vi "IMAQdx_AbsImage_Chameleon3_v5.vi"() -> ()   [LabVIEW 2015]
doc: "Take a single PixelFly exposure and display the result as an intensity graph.This VI illustrates the basics of taking an exposure with the PixelFly camera. Use Ctrl-H to get help on any of the controls\n\nCopyright 2001, The Cooke Corporation."
uses:
  Shared Libraries/Controls/FileName_Cluster.ctl
  <vilib>/userdefined/High Color/IMAQdx.ctl
  <vilib>/vision/driver/IMAQdx.llb/IMAQdx Acquisition Mode.ctl
  Shared Libraries/Controls/FileInfo_Global.vi
  <vilib>/vision/driver/NI_Vision_Acquisition_Software.lvlib
panel:
  out "DDE Done":bool=TRUE
  out "Waiting for PIXIS file":bool=TRUE
  in  "Flea Acquire":bool=TRUE
  in  "PIXIS Acquire":bool
  out "PIXIS Loop":i32
  out "CycleDone":bool
  out "PIXIS Frames":i64
  in  "Interrupt":bool
  out "Status":string="Running..."
  in  "stop":bool
  in  "Tab Control":enum32{"Setup", "Images", "Hardware status"}(tab)
  in  "PIXIS Data Series Name":string="PIXIS_Seq"
  in  "PointGrey File Parameters":T1={"Data Root"=path "D:/Data", "Index"=0, "Instrument"="Chameleon3"} {"Index" format="%04d"}
  in  "PIXIS Wave Name":string="Test_Img"
  out "PIXIS Image Note":string
  in  "Source of Control Data":refnum<k21>
  out "SPE delete path":path
  in  "PG Data Series Name":string="Chameleon3"
  in  "Camera Name":T2="Chameleon3"
  in  "Experiment":enum16{"Cs"}(ring)=4
  in  "Accept parameters from remote system":bool
  in  "PointGrey Magnification":dbl=1.0
  in  "Flea Image direction":enum16{"XY", "XZ"}(ring)=enum."XZ"
  in  "Flea Imaging technique":enum16{"Absorption", "Fluorescence", "RawImage"}(ring)
  in  "Send PG data to Igor?":bool
  out "Command to Igor":string
  out "Image note":string
  in  "PointGrey Wave Name":string="Chameleon3_Img"
  in  "Save files to archive?":bool
  out "Timeout":bool
  out "Trigger Overrun":bool
  in  "Source of File Data":refnum<k21>="\\\\Control\\VariableLibrary\\Instruction String"
  in  "Timeout (ms)":u32=20000
  in  "Gain":dbl
  in  "Shutter speed":dbl=100.0
  in  "PIXIS Magnification":dbl=1.0
  in  "PIXIS Image direction":enum16{"XY", "XZ"}(ring)
  in  "PIXIS Imaging technique":enum16{"Absorption", "Fluorescence", "RawImage"}(ring)
  in  "SPE File Path":path
  in  "Send PIXIS data to Igor?":bool
  in  "PIXIS File Parameters":T1={"Data Root"=path "I:/Data", "Index"=0, "Instrument"="PIXIS"} {"Index" format="%04d"}
  in  "Source of Wavemeter Data":refnum<k21>
  in  "Accept wavelength from remote system":bool
  in  "Flea Raw image to view":u16(ring)=1 items=["Clear", "Absorbtion", "Probe", "Background"]
  in  "Update Graphics":bool=TRUE
  out "Flea Raw Image":u16[][](graph)
  out "Flea Processed Image":sgl[][](graph)
  out "PIXIS Processed Image":sgl[][](graph)
  out "PIXIS Raw Image":u16[][](graph)
  in  "PIXIS Raw image to view":u16(ring)=1 items=["Clear", "Absorbtion", "Probe", "Background"]
  out "Camera Error":errorcluster
  out "DDE Error":errorcluster={"status"=FALSE, "code"=0, "source"="DDE Close: No Error"}
  out "Status Array":T3(array[cluster])
  in  "SPE Load Error In":errorcluster
  out "DataBlock Info":T4={"frame count"=4, "frame size"=524288, "frame stride"=524288, "N ROI"=1, "ROI widths"=[512], "ROI heights"=[512], "ROI sizes"=[524288], "ROI strides"=[524288]}
  out "DS Error":errorcluster
  out "XML Parse Errors":string
  out "Data Array Size":i32=1
  out "SPE Load Error Out":errorcluster
  out "Flea Path":path=path "D:/Data/Chameleon3temp.ibw"
  out "PIXIS Path":path=path "C:/Experiment/Data/PIXIStemp.ibw"
  out "PIXIS Images":u16[][][](array[numeric])
  out "Flea Images":u16[][][](array[numeric])
  out "Buffer Number":u32=1
  out "Flea Frames":i32
  out "Flea Loop":i32
  # "Image Acquisition v4.6 (FOR USB3 CAMERAS ONLY!!!)"
  # "Experimental Parameters"
  # "These are only get set on 1st run.\nUse a Gain of 0, Shutter Speed not used"
  # "In both techniques 3 images\nare aquired, but in Fluorescense\nthe 3rd is discarded"
  # "Obsolete: (now done with network variables)\nWhen paramaters are accepted from a remote system a DataSockets server\nmust be running on this machine (in start menu in National Instruments folder)"
  # "Camera configuration"
  # "File configuration"
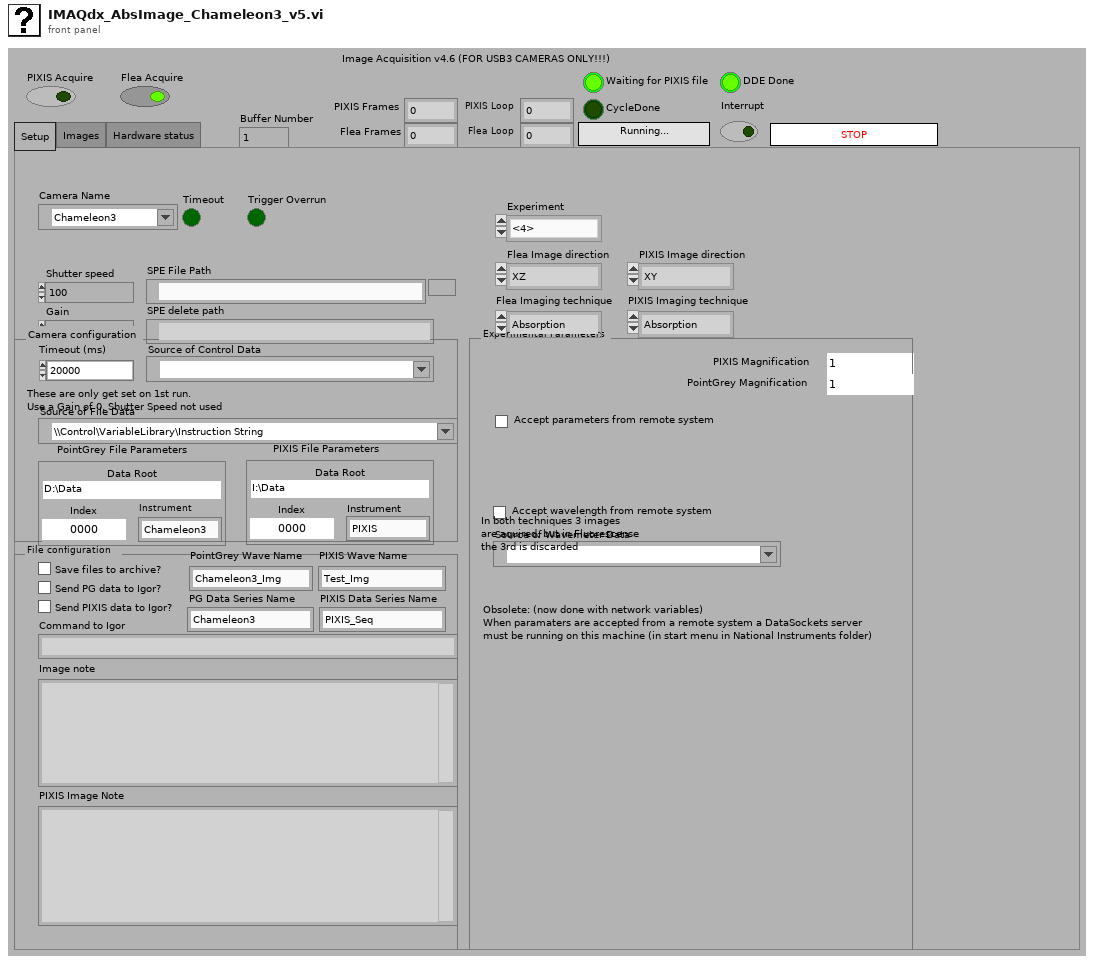
[diagram p1: front panel]
types:
  T1 = typedef "FileName_Cluster.ctl" = cluster{"Data Root":path, "Index":u32, "Instrument":string}
  T2 = typedef "IMAQdx.ctl" = refnum<k21>
  T3 = cluster{"AcquisitionInProgress":bool, "BufferCount":u32, "LastBufferNumber":u32, "LostBufferCount":u32}[]
  T4 = cluster{"frame count":i64, "frame size":i64, "frame stride":i64, "N ROI":i64, "ROI widths":i64[], "ROI heights":i64[], "ROI sizes":i64[], "ROI strides":i64[]}
  T5 = typedef "NI_Vision_Acquisition_Software.lvlib/IMAQdx Acquisition Mode.ctl" = enum32{"One Shot", "Continuous"}
  T6 = typedef "Image Type" = u32
  T7 = typedef "IMAQ Image.ctl" = refnum<image>
  T8 = cluster{"AcquisitionInProgress":bool, "BufferCount":u32, "LastBufferNumber":u32, "LostBufferCount":u32}
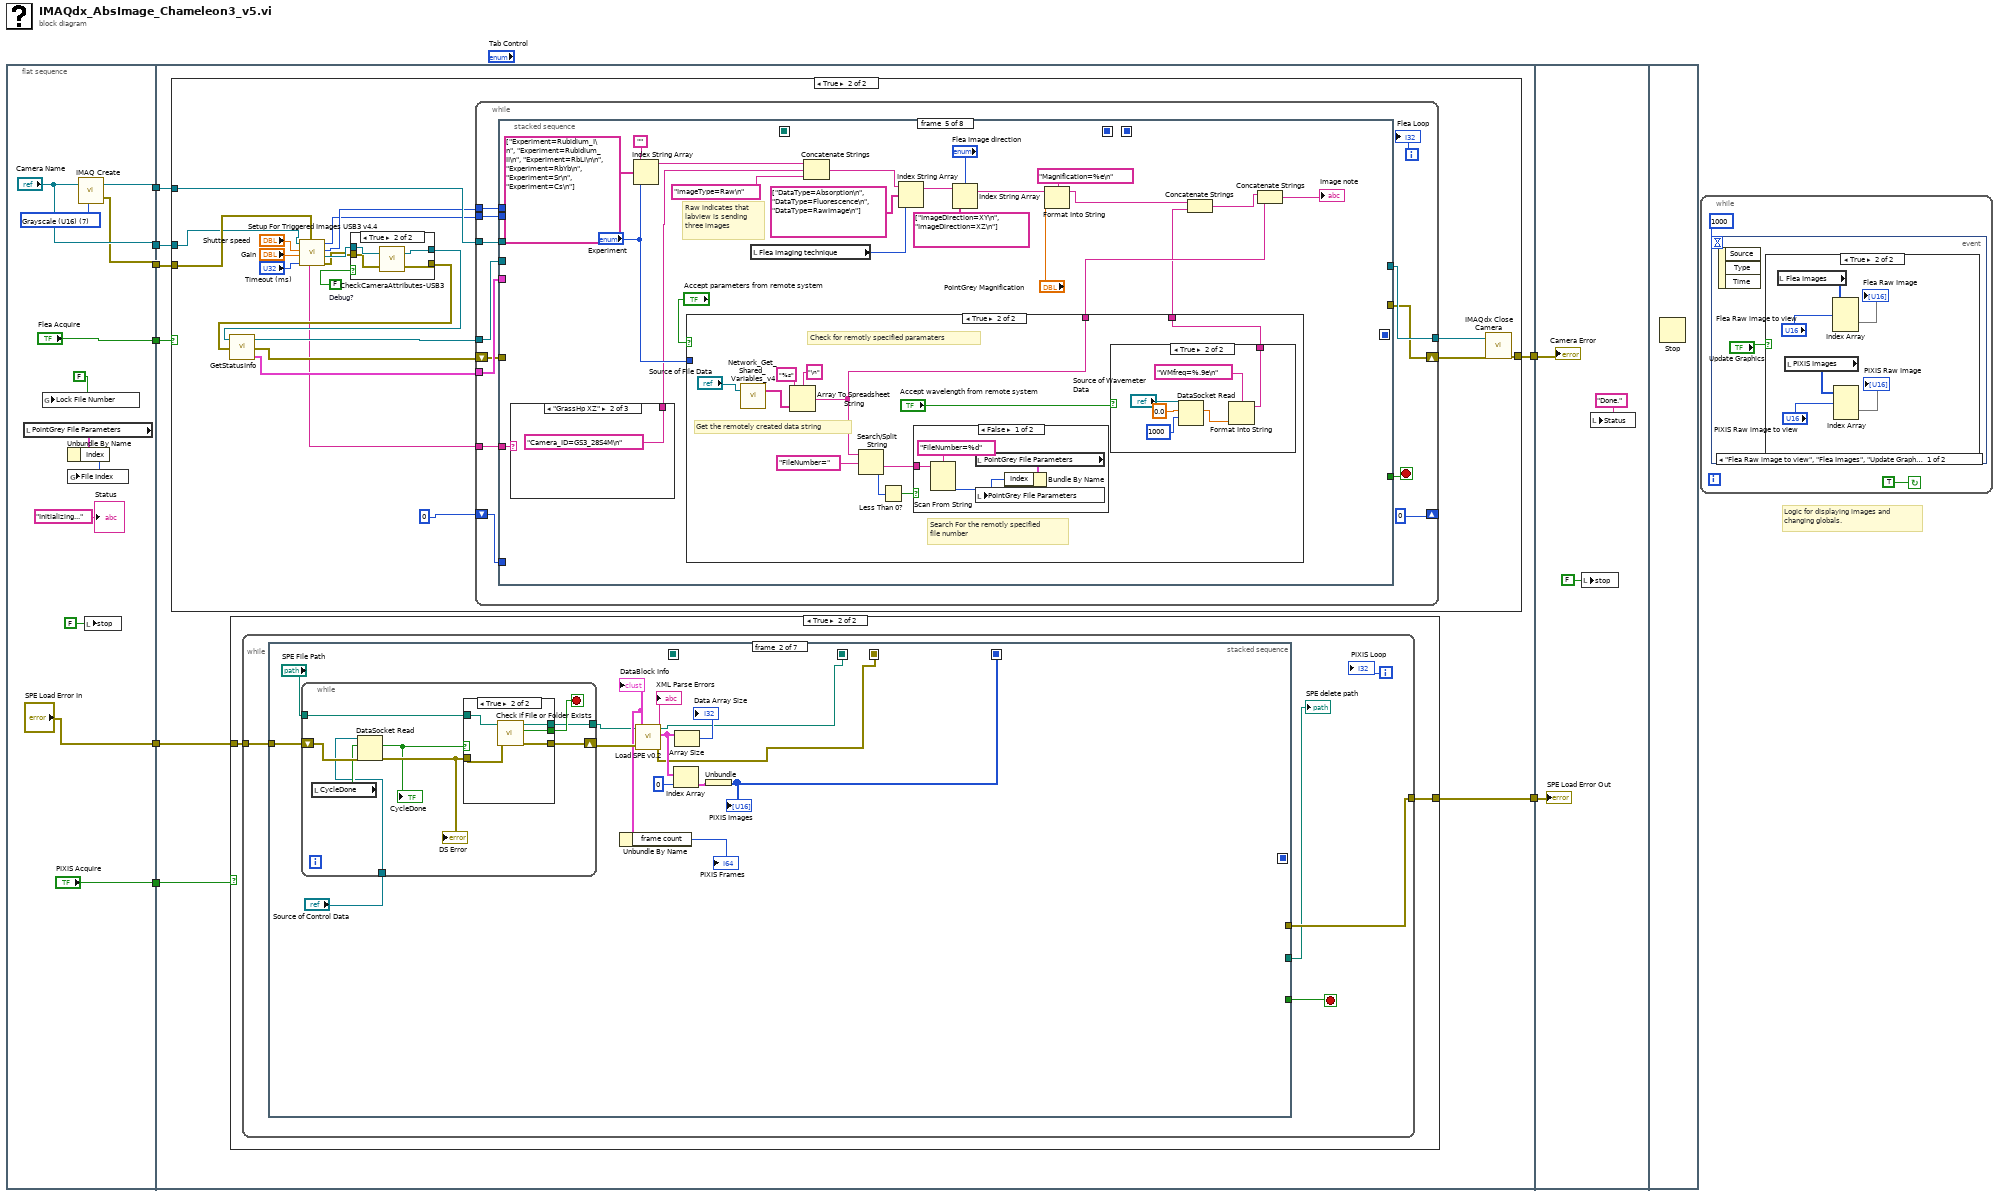
[diagram p0: block diagram]
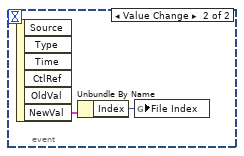
[diagram p3: hidden frame]
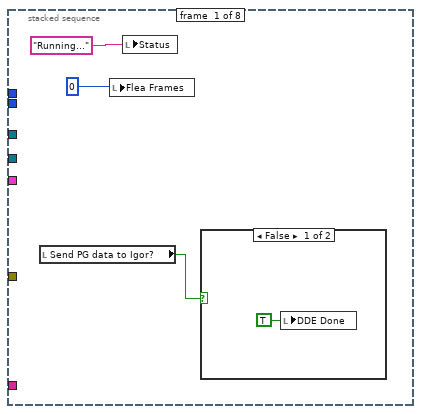
[diagram p6: hidden frame]
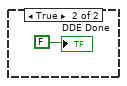
[diagram p7: hidden frame]
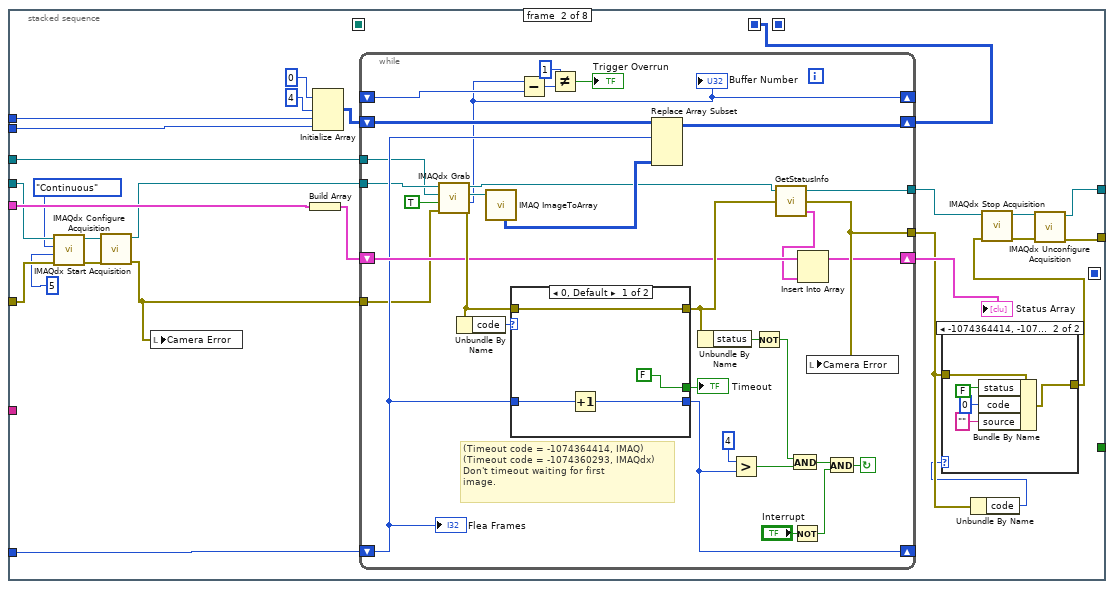
[diagram p8: hidden frame]
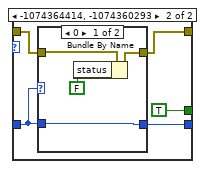
[diagram p10: hidden frame]
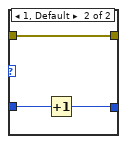
[diagram p11: hidden frame]
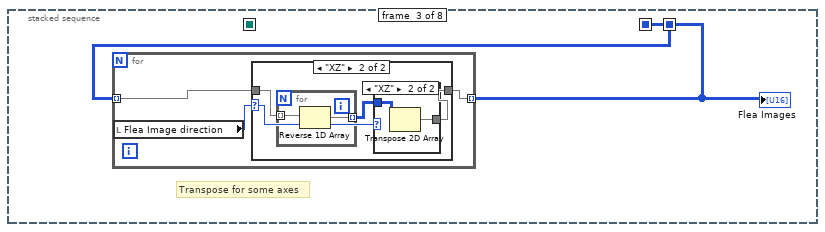
[diagram p12: hidden frame]
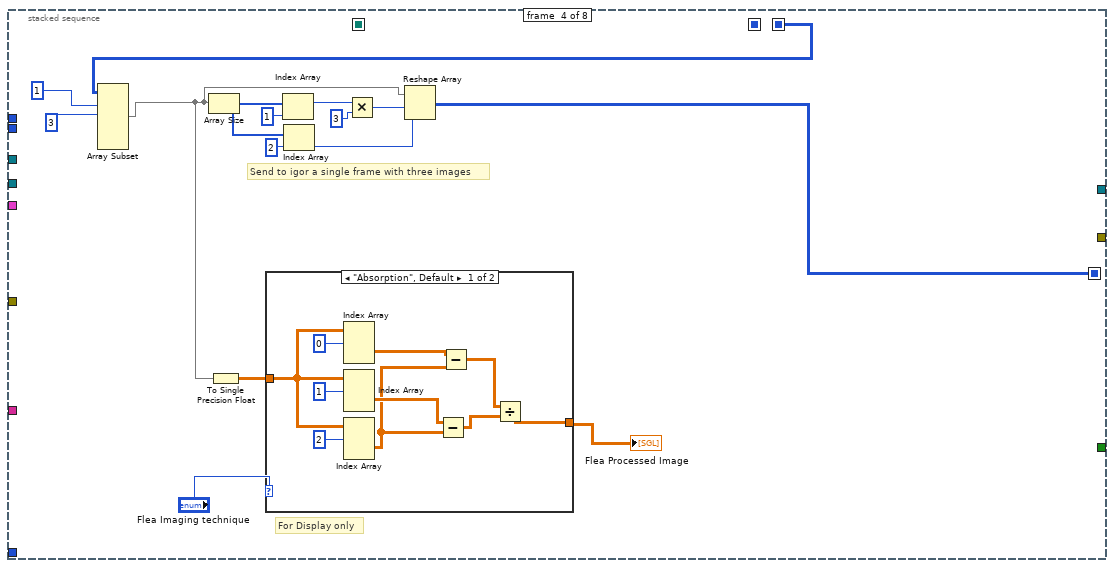
[diagram p15: hidden frame]
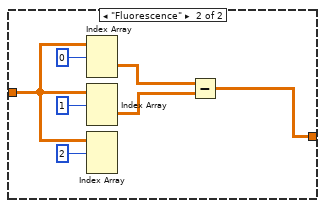
[diagram p16: hidden frame]
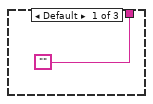
[diagram p17: hidden frame]
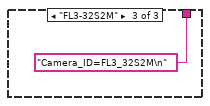
[diagram p18: hidden frame]
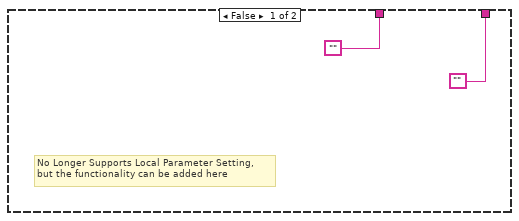
[diagram p19: hidden frame]
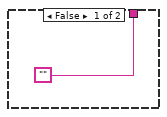
[diagram p20: hidden frame]
diagram:
  # "Logic for displaying images and\nchanging globals."
  n1 = flat-sequence {
    tunnel: [w16] -> w8
    tunnel: ["Camera Name"] -> w7
    tunnel: [w14] -> w6
    tunnel: ["SPE Load Error In"] -> w5
    tunnel: ["PIXIS Acquire"] -> w3
    tunnel: ["Flea Acquire"] -> w1
    tunnel: w7 -> [w28]
    tunnel: w8 -> [w26]
    tunnel: w6 -> [w27]
    tunnel: w5 -> [w25]
    tunnel: [w24] -> w4
    tunnel: w3 -> [w23]
    tunnel: [w22] -> w2
    tunnel: w1 -> [w21]
    tunnel: w4 -> [w473]
    tunnel: w2 -> [w472]
    frame #0 {
      w13 = T6 7 items=["Grayscale (U8)", "Grayscale (I16)", "Grayscale (SGL)", "Complex (CSG)", "RGB (U32)", "HSL (U32)", "RGB (U64)", "Grayscale (U16)"] ("Image Type")
      n2 = local read "PointGrey File Parameters"() -> (w17:T1)
      n3 = global write "FileInfo_Global.vi" "Lock File Number"(FALSE) -> ()
      n4 = Unbundle By Name(w17) -> ("Index"=w18:u32)
      n5 = global write "FileInfo_Global.vi" "File Index"(w18) -> ()
      n6 = call "IMAQ Create"("Image Name"="Camera Name", "Image Type"=w13) -> ("New Image"=w16:T7, "error out"=w14:errorcluster)  [unwired: 2 in, 1 out]
      n7 = local write "stop"(FALSE ("stop")) -> ()
      "Status" <- "Initializing..."
    }
    frame #1 {
      n8 = case shown="True" w21 {
        tunnel: w28 -> [_ w34]
        tunnel: w27 -> [w29 w35]
        tunnel: w26 -> [_ w47]
        tunnel: [w29 w44] -> w22
        frame False {
        }
        frame True {
          w50 = FALSE  # Debug?
          n9 = call "Setup For Triggered Images USB3 v4.4.vi"("error in"=w35, "Timeout"="Timeout (ms)", "Gain"="Gain", "Shutter speed"="Shutter speed", "Camera Name"=w34) -> ("Error out"=w38:errorcluster, "Session Out"=w39:T2, "Height"=w37:u32, "Width"=w36:u32, "DeviceID"=w30:string)
          n10 = case shown="True" w50 {
            tunnel: [w51 w55] -> w49
            tunnel: [w52 w54] -> w48
            tunnel: w39 -> [w51 w56]
            tunnel: w38 -> [w52 w53]
            frame False {
            }
            frame True {
              n11 = call "CheckCameraAttributes-USB3.vi"("error in"=w53, "Camera Name"=w56) -> ("error out"=w54:errorcluster, "Session Out"=w55:T2)
            }
          }
          n12 = call "GetStatusInfo.vi"("error in"=w48, "Camera In"=w49) -> ("Status Info"=w46:T8, "error out"=w43:errorcluster, "Camera Out"=w42:T2)  [unwired: 1 in]
          n13 = while {
            tunnel: w42 -> [w67]
            tunnel: w47 -> [w66]
            tunnel: w37 -> [w65]
            tunnel: w36 -> [w64]
            tunnel: w46 -> [w63]
            tunnel: [w62] -> w41
            shift-right: [0] -> _
            shift-left: 0 -> [w61]
            shift-right: [w58] -> w40
            shift-left: w43 -> [w59]
            tunnel: w30 -> [w57]
            i -> [w69]
            stop <- w68 stop-if-true
            n14 = stacked-sequence {
              seq-local: [_ _ _ w184 _ _ _ _] -> [_ _ _ _ _ w258 _ _]
              seq-local: [_ _ _ _ _ w254 _ _] -> [_ _ _ _ _ _ _ w268]
              seq-local: [_ w89 _ _ _ _ _ _] -> [_ _ w158 _ _ _ _ _]
              seq-local: [_ _ w157 _ _ _ _ _] -> [_ _ _ w175 _ _ _ _]
              tunnel: [_ _ _ _ _ _ _ "stop"] -> w68
              tunnel: w67 -> [_ w81 _ _ _ _ _ _]
              tunnel: w66 -> [_ w97 _ _ _ _ _ _]
              tunnel: w65 -> [_ w96 _ _ _ _ _ _]
              tunnel: w64 -> [_ w95 _ _ _ _ _ _]
              tunnel: w63 -> [_ w93 _ _ _ _ _ _]
              tunnel: [_ w76 _ _ _ _ _ _] -> w62
              tunnel: [_ w75 _ _ _ _ _ _] -> w58
              tunnel: w61 -> [_ w92 _ _ _ _ _ _]
              tunnel: w59 -> [_ w84 _ _ _ _ _ _]
              tunnel: w57 -> [_ _ _ _ w205 _ _ _]
              frame #0 {
                n15 = local read "Send PG data to Igor?"() -> (w70:bool)
                n16 = local write "Flea Frames"(0) -> ()
                n17 = local write "Status"("Running...") -> ()
                n18 = case shown="False" w70 {
                  frame False {
                    n19 = local write "DDE Done"(TRUE ("DDE Done")) -> ()
                  }
                  frame True {
                    "DDE Done" <- FALSE
                  }
                }
              }
              frame #1 {
                n20 = call <vilib>:"IMAQdx Configure Acquisition.vi"("error in"=w84, "Number of Buffers"=u32 5, "Continuous?"=IMAQdx_Acquisition_Mode."Continuous", "Session In"=w81) -> ("error out"=w83:errorcluster, "Session Out"=w82:T2)  [unwired: 6 in]
                n21 = call <vilib>:"IMAQdx Start Acquisition.vi"("error in"=w83, "Session In"=w82) -> ("error out"=w85:errorcluster, "Session Out"=w88:T2)  [unwired: 8 out]
                n22 = local write "Camera Error"(w85) -> ()
                n23 = Build Array(w93) -> (w94:T3)
                n24 = Initialize Array(u16 0, 4, w96, w95) -> (w99:u16[][][])
                n25 = while {
                  shift-right: [w111] -> _
                  shift-left: _ -> [w135]
                  tunnel: [w119] -> w87
                  tunnel: [w116] -> w91
                  shift-right: [w126] -> _
                  shift-left: w92 -> [w113]
                  shift-right: [w131] -> w89
                  shift-left: w99 -> [w132]
                  shift-right: [w114] -> w98
                  shift-left: w94 -> [w115]
                  tunnel: w88 -> [w110]
                  tunnel: w97 -> [w109]
                  tunnel: w85 -> [w108]
                  stop <- w122 continue-if-true
                  # "(Timeout code = -1074364414, IMAQ)\n(Timeout code = -1074360293, IMAQdx)\nDon't timeout waiting for first\nimage."
                  n26 = call <vilib>:"IMAQdx Grab.vi"("error in"=w108, "Wait for Next Buffer? (Yes)"=TRUE, "Image In"=w109, "Session In"=w110) -> ("error out"=w130:errorcluster, "Buffer Number Out"=w111:u32, "Image Out"=w125:T7, "Session Out"=w118:T2)  [unwired: 4 out]
                  "Buffer Number" <- w111
                  n27 = Unbundle By Name(w130) -> ("code"=w139:i32)
                  n28 = call "IMAQ ImageToArray"("Image"=w125) -> ("Image Pixels (U16)"=w124:u16[][])  [unwired: 2 in, 5 out]
                  n29 = case shown="0, Default" w139 {
                    tunnel: w130 -> [w144 w148]
                    tunnel: [w144 w147] -> w117
                    tunnel: [FALSE TRUE] -> w140
                    tunnel: w113 -> [w142 w146]
                    tunnel: [w141 w145] -> w126
                    frame 0, Default {
                      n30 = Increment(x=w142) -> (x+1=w141:i32)
                    }
                    frame -1074364414, -1074360293 {
                      n31 = case shown="0" w146 {
                        tunnel: [w150 w156] -> w147
                        tunnel: w148 -> [w152 w156]
                        tunnel: w146 -> [w151 w155]
                        tunnel: [w151 w154] -> w145
                        frame 0 {
                          n32 = Bundle By Name(cluster=w152, "status"=FALSE) -> (w150:errorcluster)
                        }
                        frame 1, Default {
                          n33 = Increment(x=w155) -> (x+1=w154:i32)
                        }
                      }
                    }
                  }
                  "Timeout" <- w140
                  n34 = Subtract(x=w111, y=w135) -> (x-y=w136:u32)
                  n35 = Not Equal?(x=u32 1, y=w136) -> (x != y?=→"Trigger Overrun":bool)
                  n36 = Replace Array Subset(array=w132, new element=w124, index (dim 0)=w113) -> (w131:u16[][][])  [unwired: 2 in]
                  n37 = Unbundle By Name(w117) -> ("status"=w134:bool)
                  n38 = Greater?(x=4, y=w126) -> (0:w127:bool)
                  n39 = Not(x=w134) -> (.not. x?=w133:bool)
                  n40 = call "GetStatusInfo.vi"("error in"=w117, "Camera In"=w118) -> ("Status Info"=w112:T8, "error out"=w116:errorcluster, "Camera Out"=w119:T2)  [unwired: 1 in]
                  n41 = And(x=w133, y=w127) -> (x .and. y?=w123:bool)
                  n42 = Not(x="Interrupt") -> (.not. x?=w120:bool)
                  n43 = Insert Into Array(array=w115, new element=w112) -> (w114:T3)  [unwired: 1 in]
                  n44 = local write "Camera Error"(w116) -> ()
                  n45 = And(x=w123, y=w120) -> (x .and. y?=w122:bool)
                  "Flea Frames" <- w113
                }
                "Status Array" <- w98
                n46 = Unbundle By Name(w91) -> ("code"=w90:i32)
                n47 = case shown="-1074364414, -1074360293" w90 {
                  tunnel: [w102 w106] -> w86
                  tunnel: w91 -> [w102 w105]
                  frame 0, Default {
                  }
                  frame -1074364414, -1074360293 {
                    n48 = Bundle By Name(cluster=w105, "status"=FALSE, "code"=0, "source"="") -> (w106:errorcluster)
                  }
                }
                n49 = call <vilib>:"IMAQdx Stop Acquisition.vi"("error in"=w86, "Session In"=w87) -> ("error out"=w77:errorcluster, "Session Out"=w78:T2)  [unwired: 8 in]
                n50 = call <vilib>:"IMAQdx Unconfigure Acquisition.vi"("error in"=w77, "Session In"=w78) -> ("error out"=w75:errorcluster, "Session Out"=w76:T2)  [unwired: 8 in]
              }
              frame #2 {
                # "Transpose for some axes"
                n51 = for {
                  tunnel: w158 -> [w160] mode=indexing
                  tunnel: [w159] -> w157 mode=indexing
                  n52 = local read "Flea Image direction"() -> (w161:enum16{"XY", "XZ"})
                  n53 = case shown="\"XZ\"" w161 {
                    selector: w161 -> [_ w166]
                    tunnel: w160 -> [w162 w165]
                    tunnel: [w162 w163] -> w159
                    frame Default {
                    }
                    frame "XZ" {
                      n54 = for {
                        tunnel: w165 -> [w168] mode=indexing
                        tunnel: [w167] -> w164 mode=indexing
                        n55 = Reverse 1D Array(array=w168) -> (reversed array=w167:u16[])
                      }
                      n56 = case shown="\"XZ\"" w166 {
                        tunnel: w164 -> [w169 w171]
                        tunnel: [w169 w170] -> w163
                        frame Default {
                        }
                        frame "XZ" {
                          n57 = Transpose 2D Array(2D array=w171) -> (transposed array=w170:u16[][])
                        }
                      }
                    }
                  }
                }
                "Flea Images" <- w157
              }
              frame #3 {
                # "Send to igor a single frame with three images"
                # "For Display only"
                n58 = Array Subset(array=w175, index (dim 0)=1 ("index"), length (dim 0)=3 ("length")) -> (w172:u16[][][])  [unwired: 4 in]
                n59 = Array Size(array=w172) -> (size(s)=w180:i32[])
                n60 = To Single Precision Float(number=w172) -> (single precision float=w181:sgl[][][])
                n61 = case shown="\"Absorption\", Default" "Flea Imaging technique" {
                  tunnel: [w193 w199] -> w185
                  tunnel: w181 -> [w192 w200]
                  frame "Absorption", Default {
                    n62 = Index Array(array=w192, index (dim 0)=0 ("Number of buffers")) -> (element=w191:sgl[][])  [unwired: 2 in]
                    n63 = Index Array(array=w192, index (dim 0)=1 ("Number of buffers")) -> (element=w190:sgl[][])  [unwired: 2 in]
                    n64 = Index Array(array=w192, index (dim 0)=2 ("Number of buffers")) -> (element=w189:sgl[][])  [unwired: 2 in]
                    n65 = Subtract(x=w190, y=w189) -> (x-y=w188:sgl[][])
                    n66 = Subtract(x=w191, y=w189) -> (x-y=w187:sgl[][])
                    n67 = Divide(x=w187, y=w188) -> (x/y=w193:sgl[][])
                  }
                  frame "Fluorescence" {
                    n68 = Index Array(array=w200, index (dim 0)=0 ("Number of buffers")) -> (element=w198:sgl[][])  [unwired: 2 in]
                    n69 = Index Array(array=w200, index (dim 0)=1 ("Number of buffers")) -> (element=w197:sgl[][])  [unwired: 2 in]
                    n70 = Index Array(array=w200, index (dim 0)=2 ("Number of buffers")) -> ()  [unwired: 2 in, 1 out]
                    n71 = Subtract(x=w198, y=w197) -> (x-y=w199:sgl[][])
                  }
                }
                "Flea Processed Image" <- w185
                n72 = Index Array(array=w180, index=1 ("Number of buffers")) -> (element=w177:i32)
                n73 = Index Array(array=w180, index=2 ("Number of buffers")) -> (element=w176:i32)
                n74 = Multiply(x=w177, y=3 ("Number of buffers")) -> (x*y=w182:i32)
                n75 = Reshape Array(w172, w182, w176) -> (w184:u16[][])
              }
              frame #4 {
                # "Raw indicates that\nlabview is sending\nthree images"
                n76 = case shown="\"GrassHp XZ\"" w205 {
                  tunnel: ["" "Camera_ID=GS3_28S4M\n" "Camera_ID=FL3_32S2M\n"] -> w204
                  frame Default {
                  }
                  frame "GrassHp XZ" {
                  }
                  frame "FL3-32S2M" {
                  }
                }
                n77 = Index String Array(1:"Experiment", 2:string[] ["Experiment=Rubidium_I\n", "Experiment=Rubidium_II\n", "Experiment=RbLi\n\n", "Experiment=RbYb\n", "Experiment=Sr\n", "Experiment=Cs\n"], 3:"") -> (0:w214:string)
                n78 = case shown="True" "Accept parameters from remote system" {
                  tunnel: ["" w234] -> w218
                  tunnel: "Experiment" -> [_ _]
                  tunnel: ["" w231] -> w206
                  frame False {
                    # "No Longer Supports Local Parameter Setting,\nbut the functionality can be added here"
                  }
                  frame True {
                    # "Check for remotly specified paramaters"
                    # "Get the remotely created data string"
                    # "Search For the remotly specified\nfile number"
                    n79 = call "Network_Get_Shared_Variables_v4.vi"("Source of Data"="Source of File Data") -> ("Igor Instruction String"=w241:string[])  [unwired: 1 in, 1 out]
                    n80 = Array To Spreadsheet String(delimiter (Tab)="\n", array=w241, 3:"%s") -> (spreadsheet string=w234:string)
                    n81 = Search/Split String(string=w234, search string/char (-)="FileNumber=") -> (match + rest of string=w237:string, offset of match=w236:i32)  [unwired: 2 out]
                    n82 = Less Than 0?(x=w236) -> (x < 0?=w235:bool)
                    n83 = case shown="False" w235 {
                      tunnel: w237 -> [w253 _]
                      frame False {
                        n84 = Scan From String(format string="FileNumber=%d", input string=w253) -> (output 1=w249:i32)  [unwired: 2 in, 4 out]
                        n85 = local read "PointGrey File Parameters"() -> (w251:T1)
                        n86 = Bundle By Name(cluster=w251, "Index"=w249) -> (w250:T1)
                        n87 = local write "PointGrey File Parameters"(w250) -> ()
                      }
                      frame True {
                      }
                    }
                    n88 = case shown="True" "Accept wavelength from remote system" {
                      tunnel: ["" w243] -> w231
                      frame False {
                      }
                      frame True {
                        n89 = DataSocket Read(9:1000 ("ms timeout (10000)"), 10:0.0, 11:"Source of Wavemeter Data") -> (2:w246:dbl)  [unwired: 2 in, 6 out]
                        n90 = Format Into String(format string="WMfreq=%.9e\n", w246) -> (resulting string=w243:string)  [unwired: 2 in, 1 out]
                      }
                    }
                  }
                }
                n91 = local read "Flea Imaging technique"() -> (w222:enum16{"Absorption", "Fluorescence", "RawImage"})
                n92 = Concatenate Strings(w214, w204, "ImageType=Raw\n") -> (w215:string)
                n93 = Index String Array(1:w222, 2:string[] ["DataType=Absorption\n", "DataType=Fluorescence\n", "DataType=RawImage\n"], 3:w215) -> (0:w223:string)
                n94 = Index String Array(1:"Flea Image direction", 2:string[] ["ImageDirection=XY\n", "ImageDirection=XZ\n"], 3:w223) -> (0:w225:string)
                n95 = Format Into String(format string="Magnification=%e\n", initial string=w225, "PointGrey Magnification") -> (resulting string=w207:string)  [unwired: 1 in, 1 out]
                n96 = Concatenate Strings(w207, w206) -> (w208:string)
                n97 = Concatenate Strings(w208, w218) -> (→"Image note":string)
              }
              frame #5 {
                # "Save the file as an igor binary"
                n98 = call "MakeFileName_NIST.vi"("File Parameters"="PointGrey File Parameters", "Save permanent file?"="Save files to archive?") -> ("New file parameters."=w260:T1, "Path to File"=w262:path, "path"=w261:path)
                n99 = local write "PointGrey File Parameters"(w260) -> ()
                n100 = call "RecursiveMakeDirectory.vi"("Directory to create"=w261) -> ("error out"=w264:errorcluster)  [unwired: 1 in, 1 out]
                n101 = local read "Image note"() -> (w257:string)
                n102 = Delete(path (use dialog)=w262, error in=w264) -> (deleted path=w255:path)  [unwired: 5 out]
                n103 = call "2D INT16 to Igor Binary File.vi"("Wave Data (I16)"=w258, "Wave Note (\"\")"=w257, "WaveName"="PointGrey Wave Name", "Path (default: dialog)"=w255) -> ("Path chosen"=w254:path)
              }
              frame #6 {
                # "Be sure the file is written"
                n104 = Wait (ms)(milliseconds to wait=u32 10) -> ()  [unwired: 1 out]
              }
              frame #7 {
                n105 = case shown="True" "Send PG data to Igor?" {
                  tunnel: w268 -> [_ w280]
                  tunnel: ["" w272] -> w267
                  frame False {
                  }
                  frame True {
                    n106 = local read "Send PIXIS data to Igor?"() -> (w275:bool)
                    n107 = flat-sequence {
                      tunnel: w271 -> [w281]
                      frame #0 {
                        # "Tell Igor what file to open"
                        n108 = call <vilib>:"DDE Open Conversation.vi"("topic"="Igor", "service"="Igor") -> ("error out"=w285:errorcluster, "conversation refnum"=w287:u32)  [unwired: 1 in, 5 out]
                        n109 = call <vilib>:"DDE Execute.vi"("error in (no error)"=w285, "command"=w281, "conversation refnum in"=w287) -> ("error out"=w286:errorcluster, "conversation refnum out"=w288:u32)  [unwired: 5 out]
                        n110 = call <vilib>:"DDE Close Conversation.vi"("error in (no error)"=w286, "conversation refnum"=w288) -> ("error out"=→"DDE Error":errorcluster)  [unwired: 7 out]
                      }
                      frame #1 {
                        n111 = local write "DDE Done"(TRUE ("Waiting for Flea File")) -> ()
                      }
                      frame #2 {
                        n112 = Wait (ms)(milliseconds to wait=u32 50) -> ()  [unwired: 1 out]
                      }
                    }
                    n113 = Path To String(path=w280) -> (string=w279:string)
                    n114 = Search and Replace String(replace all?=TRUE, input string=w279, search string="\\", replace string="\\\\") -> (result string=w274:string)  [unwired: 1 in, 6 out]
                    n115 = case shown="True" w275 {
                      tunnel: w274 -> [w293 w297]
                      tunnel: "PG Data Series Name" -> [w294 w300]
                      tunnel: [w291 w298] -> w272
                      tunnel: [w291 w298] -> w271
                      frame False {
                        n116 = Format Into String(format string="AutoRunV3(\"%s\",\"%s\") ", w294, w293) -> (resulting string=w291:string)  [unwired: 2 in, 1 out]
                      }
                      frame True {
                        n117 = local read "PIXIS Data Series Name"() -> (w296:string)
                        n118 = stacked-sequence {
                          tunnel: [_ w303] -> w295
                          frame #0 {
                            n119 = while {
                              stop <- w302 continue-if-true
                              n120 = local read "Waiting for PIXIS file"() -> (w302:bool)
                              n121 = Wait (ms)(milliseconds to wait=u32 5) -> ()  [unwired: 1 out]
                            }
                          }
                          frame #1 {
                            n122 = local read "PIXIS Path"() -> (w308:path)
                            n123 = Path To String(path=w308) -> (string=w304:string)
                            n124 = Search and Replace String(replace all?=TRUE, input string=w304, search string="\\", replace string="\\\\") -> (result string=w303:string)  [unwired: 1 in, 6 out]
                          }
                        }
                        n125 = Format Into String(format string="AutoRunV4(\"%s\",\"%s\",\"%s\",\"%s\") ", w300, w297, w296, w295) -> (resulting string=w298:string)  [unwired: 2 in, 1 out]
                      }
                    }
                  }
                }
                "Command to Igor" <- w267
                "Flea Path" <- w268
              }
            }
            "Flea Loop" <- w69
          }
          n126 = call <vilib>:"IMAQdx Close Camera.vi"("error in"=w40, "Session In"=w41) -> ("error out"=w44:errorcluster)  [unwired: 9 out]
        }
      }
      n127 = case shown="True" w23 {
        tunnel: w25 -> [w309 w311]
        tunnel: [w309 w310] -> w24
        frame False {
        }
        frame True {
          n128 = while {
            tunnel: [w313] -> w310
            tunnel: w311 -> [w315]
            i -> [w316]
            stop <- w314 stop-if-true
            n129 = stacked-sequence {
              seq-local: [_ _ w365 _ _ _ _] -> [_ _ _ _ w423 _ _]
              seq-local: [_ _ _ _ w419 _ _] -> [_ _ _ _ _ _ w439]
              seq-local: [_ w323 _ _ _ _ _] -> [_ _ w353 _ _ _ _]
              seq-local: [_ w321 _ _ _ _ _] -> [_ _ _ _ _ _ w433]
              seq-local: [_ w320 _ _ _ _ _] -> [_ _ _ _ _ _ w432]
              tunnel: w315 -> [_ w322 _ _ _ _ _]
              tunnel: [_ _ _ _ _ _ w434] -> w314
              tunnel: [_ _ _ _ _ _ w431] -> w313
              tunnel: [_ _ _ _ _ _ w430] -> w312
              frame #0 {
                n130 = local write "Status"("Running...") -> ()
                n131 = local write "PIXIS Frames"(i64 0) -> ()
                "Waiting for PIXIS file" <- TRUE
              }
              frame #1 {
                n132 = while {
                  tunnel: "SPE File Path" -> [w343]
                  shift-right: [w342] -> w333
                  shift-left: w322 -> [w339]
                  tunnel: [w340] -> w325
                  tunnel: "Source of Control Data" -> [w335]
                  stop <- w341 stop-if-true
                  n133 = local read "CycleDone"() -> (w338:bool)
                  n134 = DataSocket Read(8:w339, 10:w338, 11:w335) -> (0:w337:errorcluster, 2:w336:bool)  [unwired: 2 in, 5 out]
                  "CycleDone" <- w336
                  "DS Error" <- w337
                  n135 = case shown="True" w336 {
                    tunnel: w343 -> [w346 w351]
                    tunnel: [w345 w350] -> w342
                    tunnel: [FALSE ("file or folder exists?") w349] -> w341
                    tunnel: [w346 w348] -> w340
                    tunnel: w337 -> [w345 w347]
                    frame False {
                    }
                    frame True {
                      n136 = call <vilib>:"Check if File or Folder Exists.vi"("error in (no error)"=w347, "path"=w351) -> ("error out"=w350:errorcluster, "file or folder exists?"=w349:bool, "dup path"=w348:path)  [unwired: 7 in]
                    }
                  }
                }
                n137 = call "Load SPE v0.2.vi"("Error In"=w333, "File Path In"=w325) -> ("Error Out"=w320:errorcluster, "DataBlock Info"=w327:T4, "Output Stack"=w330:cluster{u16[][][]}[], "File Path Out"=w321:path, "Parse Errors"=→"XML Parse Errors":string)  [unwired: 5 in]
                "DataBlock Info" <- w327
                n138 = Unbundle By Name(w327) -> ("frame count"=→"PIXIS Frames":i64)
                n139 = Index Array(array=w330, index=0) -> (element=w328:cluster{u16[][][]})
                n140 = Array Size(array=w330) -> (size(s)=→"Data Array Size":i32)
                n141 = Unbundle(w328) -> (w323:u16[][][])
                "PIXIS Images" <- w323
              }
              frame #2 {
                # "Send to igor a single frame with three images"
                # "For Display only"
                n142 = Array Subset(array=w353, index (dim 0)=1 ("index"), length (dim 0)=3 ("length")) -> (w354:u16[][][])  [unwired: 4 in]
                n143 = Array Size(array=w354) -> (size(s)=w361:i32[])
                n144 = To Single Precision Float(number=w354) -> (single precision float=w362:sgl[][][])
                n145 = case shown="\"Absorption\", Default" "PIXIS Imaging technique" {
                  tunnel: [w372 w379] -> w352
                  tunnel: w362 -> [w373 w380]
                  frame "Absorption", Default {
                    n146 = Index Array(array=w373, index (dim 0)=0 ("Number of buffers")) -> (element=w369:sgl[][])  [unwired: 2 in]
                    n147 = Index Array(array=w373, index (dim 0)=1 ("Number of buffers")) -> (element=w367:sgl[][])  [unwired: 2 in]
                    n148 = Index Array(array=w373, index (dim 0)=2 ("Number of buffers")) -> (element=w368:sgl[][])  [unwired: 2 in]
                    n149 = Subtract(x=w367, y=w368) -> (x-y=w371:sgl[][])
                    n150 = Subtract(x=w369, y=w368) -> (x-y=w370:sgl[][])
                    n151 = Divide(x=w370, y=w371) -> (x/y=w372:sgl[][])
                  }
                  frame "Fluorescence" {
                    n152 = Index Array(array=w380, index (dim 0)=0 ("Number of buffers")) -> (element=w378:sgl[][])  [unwired: 2 in]
                    n153 = Index Array(array=w380, index (dim 0)=1 ("Number of buffers")) -> (element=w377:sgl[][])  [unwired: 2 in]
                    n154 = Index Array(array=w380, index (dim 0)=2 ("Number of buffers")) -> ()  [unwired: 2 in, 1 out]
                    n155 = Subtract(x=w378, y=w377) -> (x-y=w379:sgl[][])
                  }
                }
                "PIXIS Processed Image" <- w352
                n156 = Index Array(array=w361, index=1 ("Number of buffers")) -> (element=w358:i32)
                n157 = Index Array(array=w361, index=2 ("Number of buffers")) -> (element=w357:i32)
                n158 = Multiply(x=w358, y=3 ("Number of buffers")) -> (x*y=w363:i32)
                n159 = Reshape Array(w354, w363, w357) -> (w365:u16[][])
              }
              frame #3 {
                # "Raw indicates that\nlabview is sending\nthree images"
                n160 = local read "Accept parameters from remote system"() -> (w384:bool)
                n161 = local read "Experiment"() -> (w385:enum16{"Cs"})
                n162 = Index String Array(1:w385, 2:string[] ["Experiment=Rubidium_I\n", "Experiment=Rubidium_II\n", "Experiment=RbLi\n\n", "Experiment=RbYb\n", "Experiment=Sr\n", "Experiment=Sr\n"], 3:"") -> (0:w389:string)
                n163 = case shown="True" w384 {
                  tunnel: ["" w405] -> w394
                  tunnel: w385 -> [_ _]
                  frame False {
                    # "No Longer Supports Local Parameter Setting,\nbut the functionality can be added here"
                  }
                  frame True {
                    # "Check for remotely specified paramaters"
                    # "Get the remotely created data string"
                    # "Search For the remotly specified\nfile number"
                    n164 = local read "Source of File Data"() -> (w404:refnum<k21>)
                    n165 = call "Network_Get_Shared_Variables_v4.vi"("Source of Data"=w404) -> ("Igor Instruction String"=w412:string[])  [unwired: 1 in, 1 out]
                    n166 = Array To Spreadsheet String(delimiter (Tab)="\n", array=w412, 3:"%s") -> (spreadsheet string=w405:string)
                    n167 = Search/Split String(string=w405, search string/char (-)="FileNumber=") -> (match + rest of string=w408:string, offset of match=w407:i32)  [unwired: 2 out]
                    n168 = Less Than 0?(x=w407) -> (x < 0?=w406:bool)
                    n169 = case shown="False" w406 {
                      tunnel: w408 -> [w417 _]
                      frame False {
                        n170 = Scan From String(format string="FileNumber=%d", input string=w417) -> (output 1=w413:i32)  [unwired: 2 in, 4 out]
                        n171 = local read "PIXIS File Parameters"() -> (w415:T1)
                        n172 = Bundle By Name(cluster=w415, "Index"=w413) -> (w414:T1)
                        n173 = local write "PIXIS File Parameters"(w414) -> ()
                      }
                      frame True {
                      }
                    }
                  }
                }
                n174 = local read "PIXIS Imaging technique"() -> (w399:enum16{"Absorption", "Fluorescence", "RawImage"})
                n175 = Concatenate Strings(w389, "Camera_ID=PIXIS\n", "ImageType=Raw\n") -> (w390:string)
                n176 = Index String Array(1:w399, 2:string[] ["DataType=Absorption\n", "DataType=Fluorescence\n", "DataType=RawImage\n"], 3:w390) -> (0:w400:string)
                n177 = Index String Array(1:"PIXIS Image direction", 2:string[] ["ImageDirection=XY\n", "ImageDirection=XZ\n"], 3:w400) -> (0:w402:string)
                n178 = Format Into String(format string="Magnification=%e\n", initial string=w402, "PIXIS Magnification") -> (resulting string=w396:string)  [unwired: 1 in, 1 out]
                n179 = Concatenate Strings(w396, w394) -> (→"PIXIS Image Note":string)
              }
              frame #4 {
                # "Save the file as an igor binary"
                n180 = local read "Save files to archive?"() -> (w418:bool)
                n181 = call "MakeFileName_NIST.vi"("File Parameters"="PIXIS File Parameters", "Save permanent file?"=w418) -> ("New file parameters."=w425:T1, "Path to File"=w427:path, "path"=w426:path)
                n182 = local write "PIXIS File Parameters"(w425) -> ()
                n183 = call "RecursiveMakeDirectory.vi"("Directory to create"=w426) -> ("error out"=w428:errorcluster)  [unwired: 1 in, 1 out]
                n184 = local read "PIXIS Image Note"() -> (w422:string)
                n185 = Delete(path (use dialog)=w427, error in=w428) -> (deleted path=w420:path)  [unwired: 5 out]
                n186 = call "2D INT16 to Igor Binary File.vi"("Wave Data (I16)"=w423, "Wave Note (\"\")"=w422, "WaveName"="PIXIS Wave Name", "Path (default: dialog)"=w420) -> ("Path chosen"=w419:path)
              }
              frame #5 {
                # "Be sure the file is written"
                n187 = Wait (ms)(milliseconds to wait=u32 10) -> ()  [unwired: 1 out]
              }
              frame #6 {
                n188 = local read "Send PG data to Igor?"() -> (w435:bool)
                n189 = Not(x=w435) -> (.not. x?=w438:bool)
                n190 = And(x="Send PIXIS data to Igor?", y=w438) -> (x .and. y?=w436:bool)
                n191 = case shown="False" w436 {
                  tunnel: w439 -> [_ w463]
                  tunnel: w433 -> [w442 w452]
                  tunnel: w432 -> [w441 w453]
                  tunnel: [w443 w454] -> w431
                  tunnel: [w440 w451] -> w430
                  frame False {
                    n192 = stacked-sequence {
                      tunnel: [w447 _] -> w443
                      tunnel: w442 -> [w446 _]
                      tunnel: w441 -> [w445 _]
                      tunnel: [w444 _] -> w440
                      frame #0 {
                        n193 = local write "Waiting for PIXIS file"(FALSE ("Waiting for PIXIS file")) -> ()
                        n194 = Delete(path (use dialog)=w446, error in=w445) -> (deleted path=w444:path, error out=w447:errorcluster)  [unwired: 3 in, 1 out]
                      }
                      frame #1 {
                        n195 = while {
                          stop <- w449 stop-if-true
                          n196 = local read "DDE Done"() -> (w449:bool)
                          n197 = Wait (ms)(milliseconds to wait=u32 5) -> ()  [unwired: 1 out]
                        }
                      }
                    }
                  }
                  frame True {
                    # "Tell Igor what file to open"
                    n198 = Path To String(path=w463) -> (string=w462:string)
                    n199 = call <vilib>:"DDE Open Conversation.vi"("topic"="Igor", "service"="Igor") -> ("error out"=w467:errorcluster, "conversation refnum"=w465:u32)  [unwired: 1 in, 5 out]
                    n200 = Search and Replace String(replace all?=TRUE, input string=w462, search string="\\", replace string="\\\\") -> (result string=w458:string)  [unwired: 1 in, 6 out]
                    n201 = Format Into String(format string="AutoRunV3(\"%s\",\"%s\") ", "PIXIS Data Series Name", w458) -> (resulting string=w456:string)  [unwired: 2 in, 1 out]
                    n202 = call <vilib>:"DDE Execute.vi"("error in (no error)"=w467, "command"=w456, "conversation refnum in"=w465) -> ("error out"=w466:errorcluster, "conversation refnum out"=w464:u32)  [unwired: 5 out]
                    n203 = local write "Command to Igor"(w456) -> ()
                    n204 = call <vilib>:"DDE Close Conversation.vi"("error in (no error)"=w466, "conversation refnum"=w464) -> ("error out"=w455:errorcluster)  [unwired: 7 out]
                    n205 = local write "DDE Error"(w455) -> ()
                    n206 = Delete(path (use dialog)=w452, error in=w453) -> (deleted path=w451:path, error out=w454:errorcluster)  [unwired: 3 in, 1 out]
                  }
                }
                n207 = local read "stop"() -> (w434:bool)
                "PIXIS Path" <- w439
              }
            }
            "SPE delete path" <- w312
            "PIXIS Loop" <- w316
          }
        }
      }
    }
    frame #2 {
      n208 = local write "stop"(FALSE ("stop")) -> ()
      n209 = local write "Status"("Done.") -> ()
      "Camera Error" <- w472
      "SPE Load Error Out" <- w473
    }
    frame #3 {
      n210 = Stop() -> ()  [unwired: 1 out]
    }
  }
  n211 = while {
    stop <- TRUE continue-if-true
    n212 = event shown="[0] \"Flea Raw image to view\", \"Flea Images\", \"Update Graphics\", \"PIXIS Raw image to view\", \"PIXIS Images\": Value Change;  Timeout" {
      selector: _ -> [_ _]
      dyn-events: _ -> [_ _]
      timeout: 1000 -> [_ _]
      event "Flea Raw image to view", "Flea Images", "Update Graphics", "PIXIS Raw image to view", "PIXIS Images": Value Change; Timeout {
        n213 = event-data() -> ()  [unwired: 4 out]
        n214 = case shown="True" "Update Graphics" {
          frame False {
          }
          frame True {
            n215 = local read "Flea Images"() -> (w483:u16[][][])
            n216 = local read "PIXIS Images"() -> (w478:u16[][][])
            n217 = Index Array(array=w483, index (dim 0)="Flea Raw image to view") -> (element=→"Flea Raw Image":u16[][])  [unwired: 2 in]
            n218 = Index Array(array=w478, index (dim 0)="PIXIS Raw image to view") -> (element=→"PIXIS Raw Image":u16[][])  [unwired: 2 in]
          }
        }
      }
      event Value Change {
        n219 = event-data() -> ("NewVal"=w484:T1)  [unwired: 6 out]
        n220 = Unbundle By Name(w484) -> ("Index"=w485:u32)
        n221 = global write "FileInfo_Global.vi" "File Index"(w485) -> ()
      }
    }
  }
